vi "OpenALPR_test_Multiply.vi"(8 "error in (no error)":errorcluster, 10 "multiplier":dbl, 11 "multiplicand":dbl) -> (0 "error out":errorcluster, 3 "product":dbl)   [LabVIEW 2014, in "OpenALPR in LabView.lvlib"]
doc: "Do a multiplication for test purpose.\n\n\n\n\nextern \"C\" void __declspec(dllexport) test_Multiple(double a, double b, double *x);"
uses:
  OpenALPR in LabView.lvlib
  Dlls/OALPRLabVIEW.dll
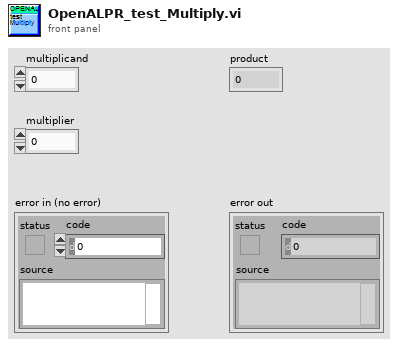
[diagram p1: front panel]
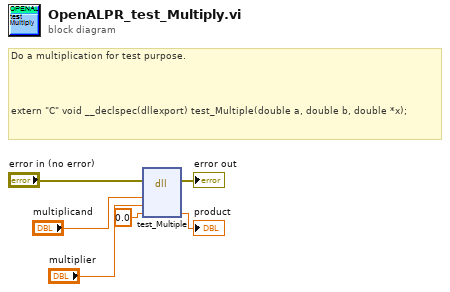
[diagram p0: block diagram]
diagram:
  # "Do a multiplication for test purpose.\n\n\n\n\nextern \"C\" void __declspec(dllexport) test_Multiple(double a, double b, double *x);"
  n1 = dll-call lib="PTH2abs EFelhasznÃ¡lÃ³kPixelbetyÃ¡rDesktopC19 -C3 Verseny bekÃ¼ldÃ©shez\tSmartMarkOpenALPR to LVOpenALPR_LabVIEWDllsOALPRLabVIEW.*" fn="test_Multiple"(error in="error in (no error)", "multiplicand"="multiplicand", "multiplier"="multiplier", "product"=0.0) -> (error out=→"error out":errorcluster, "product"=→"product":dbl)  [unwired: 5 in, 1 out]
